vi "lab2.vi"() -> ()   [LabVIEW 2015]
uses:
  <vilib>/Analysis/polynomials.llb/Scalar Polynomial Evaluation (DBL).vi
  <vilib>/ptbypt/NI_PtbyPt.lvlib
  <vilib>/Analysis/NI_AALPro.lvlib
panel:
  out "Running":bool
  in  "stop 2":bool
  in  "P(x)":dbl[](array[numeric])=[8.0, -2.0, 0.02] format="%#.10f"
  out "Celcius":dbl format="%0.3f"
  out "Waveform Chart 3":dynamicdata(graph) caption="Waveform Chart 2"
  out "Waveform Chart 2":dynamicdata(graph)
  in  "stop":bool
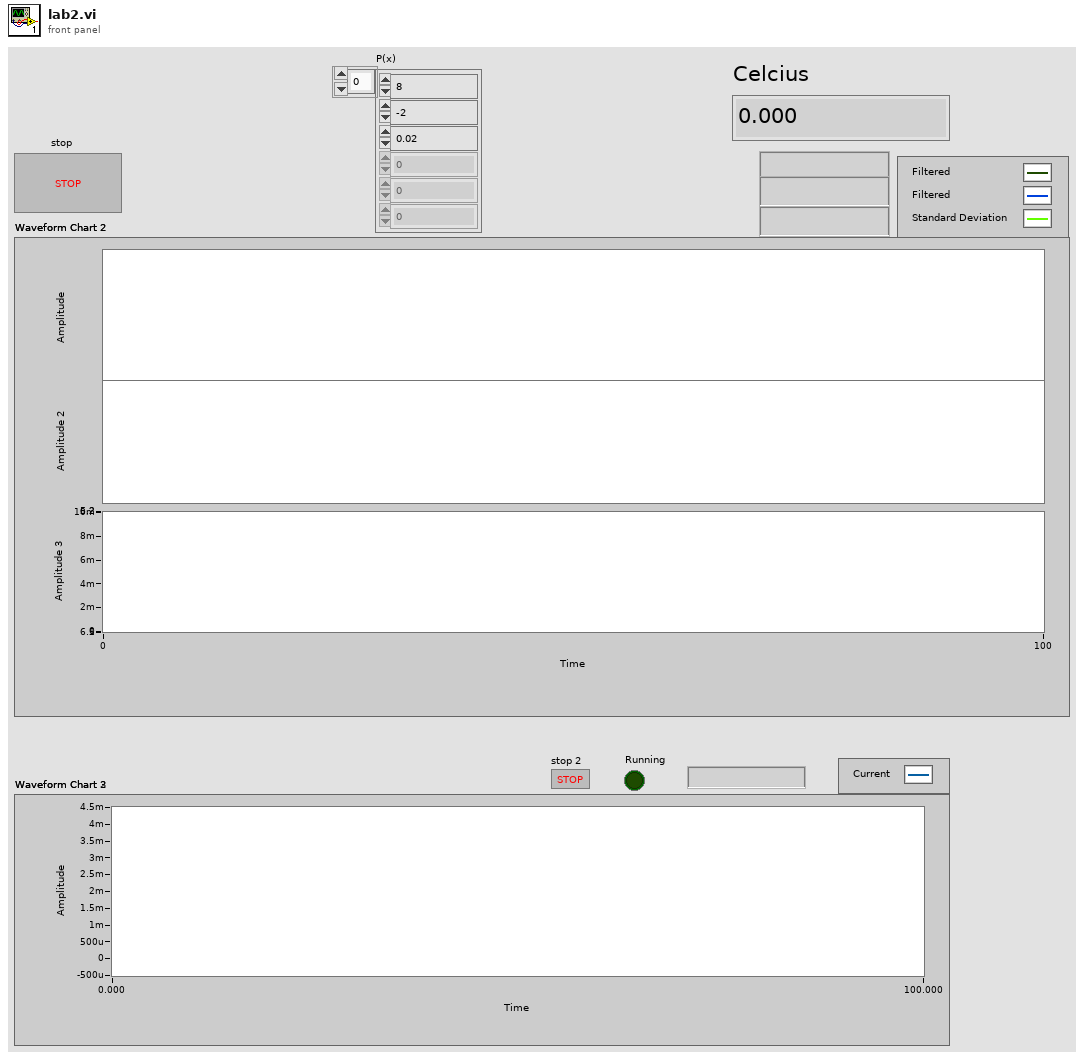
[diagram p1: front panel]
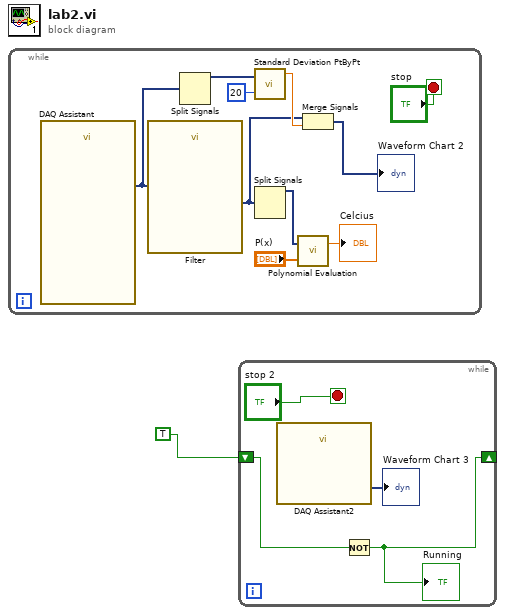
[diagram p0: block diagram]
diagram:
  n1 = while {
    stop <- "stop" stop-if-true
    n2 = call "DAQ Assistant"() -> ("data"=w2:dynamicdata)  [unwired: 17 in, 2 out]
    n3 = call "Filter"("Signal"=w2) -> ("Filtered Signal"=w9:dynamicdata)  [unwired: 9 in, 1 out]
    n4 = Split Signals(w2) -> (w4:dynamicdata)  [unwired: 4 in, 3 out]
    n5 = call <vilib>:"Standard Deviation PtByPt.vi"("x"=w4, "sample length"=20) -> ("standard deviation"=w11:dbl)  [unwired: 1 in, 2 out]
    n6 = Split Signals(w9) -> (w8:dynamicdata)  [unwired: 4 in, 3 out]
    n7 = call-poly <vilib>:"Polynomial Evaluation.vi"("P(x)"="P(x)", "a"=w8) -> ("P(a)"=→"Celcius":dbl)  [unwired: 1 out]
    n8 = Merge Signals(w9, w11) -> (→"Waveform Chart 2":dynamicdata)
  }
  n9 = while {
    shift-right: [w12] -> _
    shift-left: TRUE -> [w14]
    stop <- "stop 2" stop-if-true
    n10 = call "DAQ Assistant2"() -> ("data"=→"Waveform Chart 3":dynamicdata)  [unwired: 17 in, 2 out]
    n11 = Not(x=w14) -> (.not. x?=w12:bool)
    "Running" <- w12
  }
